vi "Delay_DMM2831E.vi"(2 "error in (no error)":errorcluster, 3 "Delay Time (0)":u32 max=5000, 4 "Instrument In":refnum<visa-resource-name>) -> (0 "error out":errorcluster, 1 "Instrument Out":refnum<visa-resource-name>)   [LabVIEW 2023]
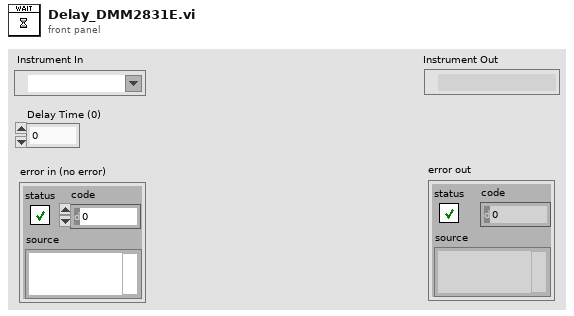
[diagram p1: front panel]
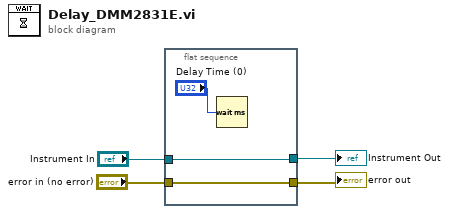
[diagram p0: block diagram]
diagram:
  n1 = flat-sequence {
    tunnel: [w6] -> w1
    tunnel: "Instrument In" -> [w6]
    tunnel: [w5] -> w2
    tunnel: "error in (no error)" -> [w5]
    frame #0 {
      n2 = Wait (ms)(milliseconds to wait="Delay Time (0)") -> ()  [unwired: 1 out]
    }
  }
  "Instrument Out" <- w1
  "error out" <- w2
